vi "carMimic.vi"() -> ()   [LabVIEW 2019]
panel:
  out "Car?":bool
  in  "CAR":bool
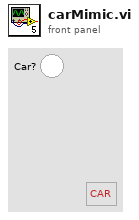
[diagram p1: front panel]
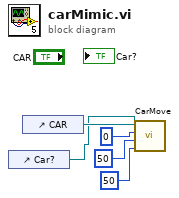
[diagram p0: block diagram]
diagram:
  n1 = control-ref of="Car?"() -> (w1:refnum<vi>)
  n2 = control-ref of="CAR"() -> (w5:refnum<vi>)
  n3 = call "CarMove.vi"("X done?"=w1, "X+Y"=50, "X"=50, "speed"=u32 0, "Boolean in"=w5) -> ()  [unwired: 7 in]
